vi "tdms test.vi"() -> ()   [LabVIEW 2013, in "Binary logger tests.lvlib"]
uses:
  Binary logger tests.lvlib
  configuration/Binary datalogger configuration.lvclass
  execution/Binary datalogger runtime.lvclass
  <vilib>/NI/Tag Bus Module Framework/channel/channel classification.ctl
  <vilib>/NI/Tag Bus/tag/Data Type.ctl
  <vilib>/Utility/sysdir.llb/System Directory Type.ctl
  <vilib>/Platform/TimedLoop/XDataNode/timing_clust.ctl
  <vilib>/Platform/TimedLoop/XDataNode/nitl_modes.ctl
  <vilib>/Platform/TimedLoop/XDataNode/wakeup.ctl
  configuration/Binary datalogger configuration.lvclass/Binary datalogger configuration.ctl
  <vilib>/NI/Tag Bus/table/data polymorphs/write one/write Boolean.vi
  configuration/Write Path.vi
  configuration/Write queue size.vi
  configuration/Write scans per write.vi
  configuration/Write backup directory.vi
  configuration/Write add enable channel.vi
  <vilib>/platform/TimedLoop/XDataNode/XDataNode.xnode
  <vilib>/NI/Tag Bus Module Framework/channel/TBM channel.lvclass
  <vilib>/NI/Tag Bus/tag/tag descriptor.lvclass
  <vilib>/NI/Tag Bus/table/data table.lvlib
  <vilib>/Platform/TimedLoop/XDataNode/XDNodeRunTimeDep.lvlib
  <vilib>/NI/Configuration Framework/serializable configuration/NISE_CEF_serializable configuration.lvclass
  <vilib>/Utility/RT CPU pool selections.ctl
panel:
  out "max":dbl
  out "min":dbl
  in  "enable state":bool=TRUE
  out "found?":bool
  in  "stop":bool
  out "error out":errorcluster
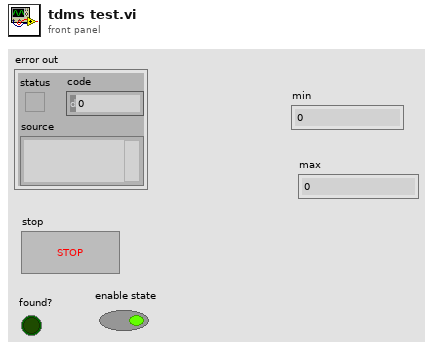
[diagram p1: front panel]
types:
  T1 = typedef "System Directory Type.ctl" = i32
  T2 = typedef "tag bus.lvlib/tag descriptor.lvclass/Data Type.ctl" = enum16{"Double", "Single", "I64", "I32", "I16", "I8", "U64", "U32", "U16", "U8", "Boolean", "String", "Array of Double", "Array of Single", "Array of I64", "Array of I32", "Array of I16", "Array of I8", "Array of U64", "Array of U32", "Array of U16", "Array of U8", "Array of Boolean", "Array of String"}
  T3 = typedef "TBM channel.lvclass/channel classification.ctl" = enum16{"input data", "output data", "processing parameter", "processing result"}
  T4 = typedef "NI_Real-Time Target Support.lvlib/RT CPU pool selections.ctl" = enum16{"System & Timed Structures", "System", "Timed Structures", "Reserved"}
  T5 = typedef "TBM channel.lvclass/data tables.ctl" = cluster{"input data":T6, "processing parameter":T6, "processing result":T6, "output data":T6}
  T6 = typedef "tag bus.lvlib/dictionary table pair.ctl" = cluster{"data dictionary":refnum<class "data dictionary.lvclass">, "data table":T7}
  T7 = typedef "tag bus.lvlib/data table.lvlib/data table.ctl" = cluster{"Double":dbl[], "Single":sgl[], "I64":i64[], "I32":i32[], "I16":i16[], "I8":i8[], "U64":u64[], "U32":u32[], "U16":u16[], "U8":u8[], "Boolean":bool[], "String":string[], "Array of Double":cluster{"DBL Array":dbl[]}[], "Array of Single":cluster{"SGL Array":sgl[]}[], "Array of I64":cluster{"I64 Array":i64[]}[], "Array of I32":cluster{"I32 Array":i32[]}[], "Array of I16":cluster{"I16 Array":i16[]}[], "Array of I8":cluster{"I8 Array":i8[]}[], "Array of U64":cluster{"U64 Array":u64[]}[], "Array of U32":cluster{"U32 Array":u32[]}[], "Array of U16":cluster{"U16 Array":u16[]}[], "Array of U8":cluster{"U8 Array":u8[]}[], "Array of Boolean":cluster{"Boolean Array":bool[]}[], "Array of String":cluster{"String Array":string[]}[]}
  T8 = typedef "XDNodeRunTimeDep.lvlib/timing_clust.ctl" = cluster{"Expected End [f-1]":u64, "Actual End [f-1]":u64, "Finished Late? [f-1]":bool, "Expected End [i-1]":u64, "Actual End [i-1]":u64, "Finished Late? [i-1]":bool, "Expected Start [i]":u64, "Actual Start [i]":u64, "Expected Start [f]":u64, "Actual Start [f]":u64, "Source Name":string, "Structure Name":string, "Period":i64, "Deadline":i64, "Offset":i64, "Start":i64, "Priority":i32, "Timeout":i32, "Mode":T9, "Wakeup Reason":T10, "Error":errorcluster, "Source Type":string, "Secondary Source Type":string, "Global End Time":u64, "Global Start Time":u64, "Frame Duration":u64, "Iteration Duration":u64, "Assigned CPU":i32, "I/O Scan Engine Mode":u32}
  T9 = typedef "XDNodeRunTimeDep.lvlib/nitl_modes.ctl" = enum32{"No Change", "Process missed periods, maintain original phase", "Discard missed periods, maintain original phase", "Process missed periods, ignore original phase", "Discard missed periods, ignore original phase"}
  T10 = typedef "XDNodeRunTimeDep.lvlib/wakeup.ctl" = enum32{"Normal", "Aborted", "Asynchronous wakeup", "Timing source error", "Timed loop error", "Timeout"}
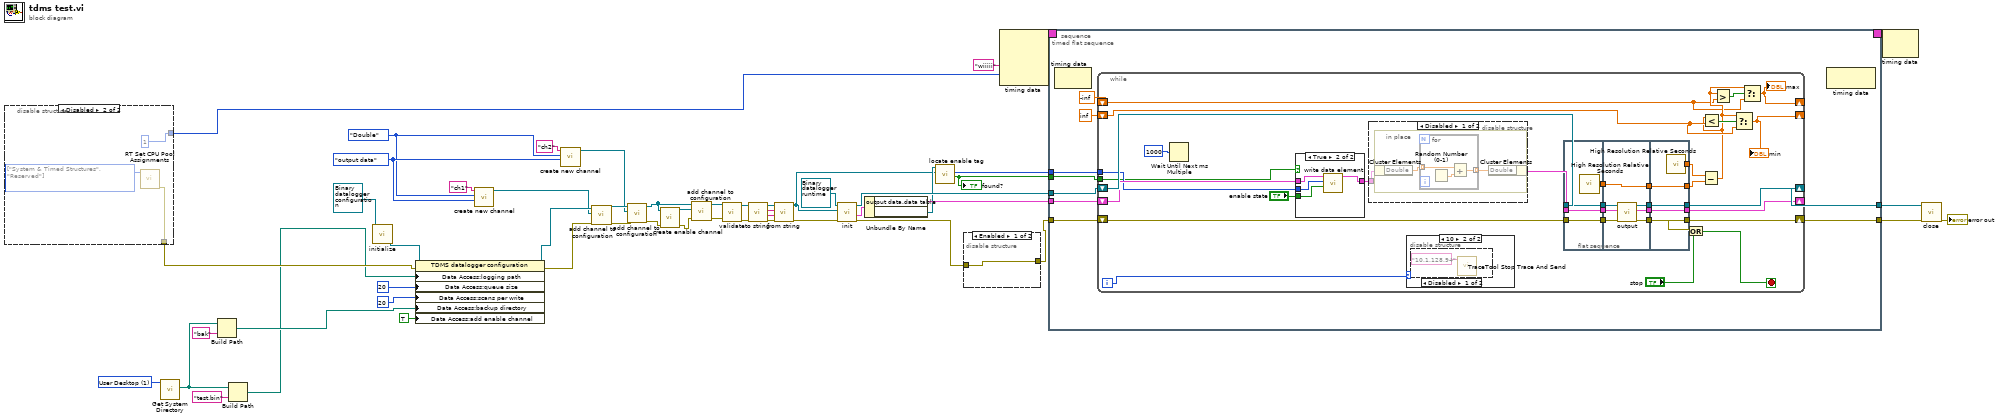
[diagram p0: block diagram]
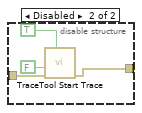
[diagram p2: hidden frame]
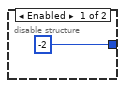
[diagram p3: hidden frame]
diagram:
  w6 = T1 1 items=["User Home"=0, "User Desktop"=1, "User Documents"=2, "User Application Data"=3, "User Preferences"=4, "User Temporary"=5, "Public Documents"=6, "Public Application Data"=7, "Public Preferences"=8, "Public Cache"=13, "System Core Libraries"=9, "System Installed Libraries"=10, "Application Files"=11, "Boot Volume Root"=12] ("system directory type")
  w36 = Data_Type."Double" ("data type")
  w37 = channel_classification."output data" ("channel classification")
  n1 = disable-structure shown="Disabled" {
    disable-tunnel: [_ w55] -> w25
    disable-tunnel: [-2 ("Processor") 1 ("Processor")] -> w24
    frame Enabled {
    }
    frame Disabled {
      w56 = T4[] [enum."System & Timed Structures", enum."Reserved"] items=["System & Timed Structures", "System", "Timed Structures", "Reserved"] ("CPU pools")
      n2 = call <vilib>:"RT Set CPU Pool Assignments.vi"("CPU pools"=w56) -> ("error out"=w55:errorcluster)  [unwired: 7 in, 3 out]
    }
  }
  n3 = call <vilib>:"Get System Directory.vi"("system directory type"=w6) -> ("system directory"=w3:path)  [unwired: 10 in]
  n4 = Build Path(base path=w3, name or relative path="bak") -> (appended path=w2:path)
  n5 = Build Path(base path=w3, name or relative path="test.bin") -> (appended path=w1:path)
  n6 = call <vilib>:"initialize.vi"("configuration in"=refnum<class "Binary datalogger configuration.lvclass"> refnum ("TDMS datalogger configuration")) -> ("configuration out"=w7:refnum<class "Binary datalogger configuration.lvclass">)  [unwired: 8 in, 2 out]
  n7 = property class="TDMS datalogger configuration"(reference=w7, error in=w25, "Data Access:logging path"=w1, "Data Access:queue size"=20 ("queue size"), "Data Access:scans per write"=20 ("scans per write"), "Data Access:backup directory"=w2, "Data Access:add enable channel"=TRUE ("add enable channel")) -> (reference out=w17:refnum<class "Binary datalogger configuration.lvclass">, error out=w16:errorcluster)
  n8 = call <vilib>:"create new channel.vi"("channel classification"=w37, "data type"=w36, "channel name"="ch1") -> ("channel"=w15:refnum<class "TBM channel.lvclass">)  [unwired: 8 in]
  n9 = call <vilib>:"create new channel.vi"("channel classification"=w37, "data type"=w36, "channel name"="ch2") -> ("channel"=w13:refnum<class "TBM channel.lvclass">)  [unwired: 8 in]
  n10 = call "add channel to configuration.vi"("error in"=w16, "TBM channel in"=w15, "bin datalogger configuration in"=w17) -> ("error out"=w14:errorcluster, "bin datalogger configuration out"=w18:refnum<class "Binary datalogger configuration.lvclass">)  [unwired: 7 in]
  n11 = call "add channel to configuration.vi"("error in"=w14, "TBM channel in"=w13, "bin datalogger configuration in"=w18) -> ("error out"=w10:errorcluster, "bin datalogger configuration out"=w9:refnum<class "Binary datalogger configuration.lvclass">)  [unwired: 7 in]
  n12 = call "create enable channel.vi"("error in"=w10, "bin datalogger configuration"=w9) -> ("error out"=w11:errorcluster, "enable channel"=w12:refnum<class "TBM channel.lvclass">)  [unwired: 7 in, 1 out]
  n13 = call "add channel to configuration.vi"("error in"=w11, "TBM channel in"=w12, "bin datalogger configuration in"=w9) -> ("error out"=w20:errorcluster, "bin datalogger configuration out"=w19:refnum<class "Binary datalogger configuration.lvclass">)  [unwired: 7 in]
  n14 = call-dynamic "validate.vi"("error in"=w20, "bin datalogger configuration in"=w19) -> ("error out"=w52:errorcluster, "bin datalogger configuration out"=w51:refnum<class "Binary datalogger configuration.lvclass">)  [unwired: 8 in]
  n15 = call-dynamic "to string.vi"("error in"=w52, "bin datalogger configuration in"=w51) -> ("error out"=w49:errorcluster, "data"=w48:string, "version"=w47:string, "bin datalogger configuration out"=w50:refnum<class "Binary datalogger configuration.lvclass">)  [unwired: 6 in]
  n16 = call-dynamic "from string.vi"("error in"=w49, "data"=w48, "version"=w47, "bin datalogger configuration in"=w50) -> ("error out"=w46:errorcluster, "bin datalogger configuration out"=w8:refnum<class "Binary datalogger configuration.lvclass">)  [unwired: 6 in]
  n17 = call-dynamic "init.vi"("error in"=w46, "TBM module configuration in"=w8, "bin datalogger runtime in"=refnum<class "Binary datalogger runtime.lvclass"> refnum ("TDMS datalogger runtime")) -> ("error out"=w23:errorcluster, "data allocations"=w38:T5, "bin datalogger runtime out"=w45:refnum<class "Binary datalogger runtime.lvclass">)  [unwired: 5 in, 1 out]
  n18 = Unbundle By Name(w38) -> ("output data.data table"=w44:T7, "output data.data dictionary"=w30:refnum<class "data dictionary.lvclass">)
  n19 = call "locate enable tag.vi"("bin datalogger configuration"=w8, "data dictionary in"=w30) -> ("found?"=w28:bool, "index"=w29:i32)  [unwired: 7 in, 1 out]
  "found?" <- w28
  n20 = disable-structure shown="Enabled" {
    disable-tunnel: [w57 w60] -> w22
    disable-tunnel: w23 -> [w57 w61]
    frame Enabled {
    }
    frame Disabled {
      n21 = call <vilib>:"TraceTool Start Trace.vi"("Detailed Tracing? (F)"=TRUE, "error in (no error)"=w61, "VI Tracing? (T)"=FALSE) -> ("error out"=w60:errorcluster)  [unwired: 7 in, 1 out]
    }
  }
  n22 = node-c288("wiiiii" ("Structure Name"), w24) -> (w27:T8)  [unwired: 2 in]
  n23 = timed-sequence {
    timing: w27 -> [_]
    timing-out: [_] -> w26
    tunnel: w45 -> [w68]
    tunnel: w22 -> [w67]
    tunnel: w44 -> [w66]
    tunnel: [w65] -> w43
    tunnel: [w64] -> w42
    tunnel: w29 -> [w63]
    tunnel: w28 -> [w62]
    n24 = timed-flat-sequence {
      tunnel: w68 -> [w77]
      tunnel: w67 -> [w76]
      tunnel: w66 -> [w75]
      tunnel: [w74] -> w65
      tunnel: [w73] -> w64
      tunnel: w63 -> [w72]
      tunnel: w62 -> [w71]
      n25 = node-c288() -> ()  [unwired: 1 in, 1 out]
      n26 = while {
        shift-right: [w97] -> w73
        shift-left: w76 -> [w108]
        shift-right: [w107] -> w74
        shift-left: w77 -> [w109]
        shift-right: [w105] -> _
        shift-left: w75 -> [w102]
        tunnel: w72 -> [w100]
        tunnel: w71 -> [w99]
        shift-right: [w80] -> _
        shift-left: -inf -> [w82]
        shift-right: [w81] -> _
        shift-left: inf -> [w84]
        i -> [w79]
        stop <- w98 stop-if-true
        n27 = Wait Until Next ms Multiple(millisecond multiple=u32 1000) -> ()  [unwired: 1 out]
        n28 = case shown="True" w99 {
          tunnel: w102 -> [w110 w114]
          tunnel: [w110 w113] -> w101
          tunnel: w100 -> [_ w112]
          tunnel: "enable state" -> [_ w111]
          frame False {
          }
          frame True {
            n29 = call-poly <vilib>:"write data element.vi"("value"=w111, "index"=w112, "data table in"=w114) -> ("data table out"=w113:T7)  [unwired: 8 in]
          }
        }
        n30 = disable-structure shown="Disabled" {
          disable-tunnel: [w133 w139] -> w106
          disable-tunnel: w101 -> [w132 w139]
          frame Disabled {
            n31 = in-place {
              n32 = in-place-cluster #1(w132) -> ("Double"=w135:dbl[])
              n33 = for {
                tunnel: w135 -> [w138] mode=indexing
                tunnel: [w137] -> w134 mode=indexing
                n34 = Random Number (0-1)() -> (number: 0 to 1=w136:dbl)
                n35 = Add(x=w138, y=w136) -> (x+y=w137:dbl)
              }
              n36 = in-place-cluster #1("Double"=w134) -> (w133:T7)
            }
          }
          frame Enabled {
          }
        }
        n37 = case shown="10" w79 {
          frame 0, Default {
          }
          frame 10 {
            n38 = disable-structure shown="Disabled" {
              frame Disabled {
                n39 = call <vilib>:"TraceTool Stop Trace And Send.vi"("Trace Host Network Address"="10.1.128.94") -> ()  [unwired: 10 in, 1 out]
              }
              frame Enabled {
              }
            }
          }
        }
        n40 = flat-sequence {
          tunnel: w106 -> [w117]
          tunnel: w108 -> [w118]
          tunnel: w109 -> [w119]
          tunnel: [w119] -> w93
          tunnel: [w118] -> w92
          tunnel: [w117] -> w91
          tunnel: [w116] -> w89
          tunnel: [w124] -> w96
          tunnel: [w122] -> w95
          tunnel: [w121] -> w94
          tunnel: w93 -> [w126]
          tunnel: w92 -> [w125]
          tunnel: w91 -> [w123]
          tunnel: [w120] -> w90
          tunnel: w89 -> [w120]
          tunnel: [w129] -> w97
          tunnel: [w130] -> w105
          tunnel: [w131] -> w107
          tunnel: w96 -> [w131]
          tunnel: w95 -> [w130]
          tunnel: w94 -> [w129]
          tunnel: [w128] -> w88
          tunnel: w90 -> [w128]
          tunnel: [w127] -> w87
          frame #0 {
            n41 = call <vilib>:"High Resolution Relative Seconds.vi"() -> ("relative seconds"=w116:dbl)
          }
          frame #1 {
            n42 = call-dynamic "output.vi"("error in"=w125, "data table in"=w123, "bin datalogger runtime in"=w126) -> ("error out"=w121:errorcluster, "data table out"=w122:T7, "bin datalogger runtime out"=w124:refnum<class "Binary datalogger runtime.lvclass">)  [unwired: 6 in]
          }
          frame #2 {
            n43 = call <vilib>:"High Resolution Relative Seconds.vi"() -> ("relative seconds"=w127:dbl)
          }
        }
        n44 = Or(x=w97, y="stop") -> (x .or. y?=w98:bool)
        n45 = Subtract(x=w87, y=w88) -> (x-y=w83:dbl)
        n46 = Less?(x=w83, y=w84) -> (x < y?=w85:bool)
        n47 = Greater?(x=w83, y=w82) -> (0:w86:bool)
        n48 = Select(t=w83, s=w85, f=w84) -> (s? t:f=w81:dbl)
        "min" <- w81
        n49 = Select(t=w83, s=w86, f=w82) -> (s? t:f=w80:dbl)
        "max" <- w80
      }
      n50 = node-c288() -> ()  [unwired: 1 in, 1 out]
    }
  }
  n51 = node-c288(w26) -> ()  [unwired: 1 out]
  n52 = call-dynamic "close.vi"("error in"=w42, "bin datalogger runtime in"=w43) -> ("error out"=→"error out":errorcluster)  [unwired: 9 in]
